vi "Add Data Tree.vi"(8 "error in (no error)":errorcluster, 11 "[V]System Tree View in":refnum<class "[V]System Tree View.lvclass">) -> (0 "error out":errorcluster, 3 "[V]System Tree View out":refnum<class "[V]System Tree View.lvclass">)   [LabVIEW 2020]
uses:
  <vilib>/HUASUI/Tree/Item/Type Definitions/Item Map.ctl
  <vilib>/HUASUI/Tree/Item/Item.lvclass
  <vilib>/HUASUI/Tree/Tree Helper/Tree Helper.lvclass
  <vilib>/HUASUI/Tree/Tree Helper.lvlib
  Models/Data List/Data List.lvclass
  [V]System Tree View.lvclass
  C:/Program Files (x86)/National Instruments/LabVIEW 2020/vi.lib/ActorFramework/Actor/Actor.lvclass
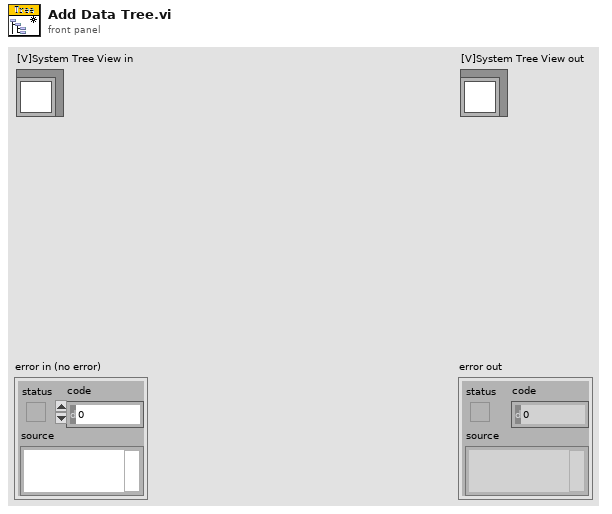
[diagram p1: front panel]
types:
  T1 = typedef "Tree Helper.lvlib/Item.lvclass/Item Map.ctl" = cluster{"Self Tag":string, "Parent Tag":string, "LeftCell Value":string, "RightCells Value":string[], "Is Child":bool, "Symbol Index":i32}
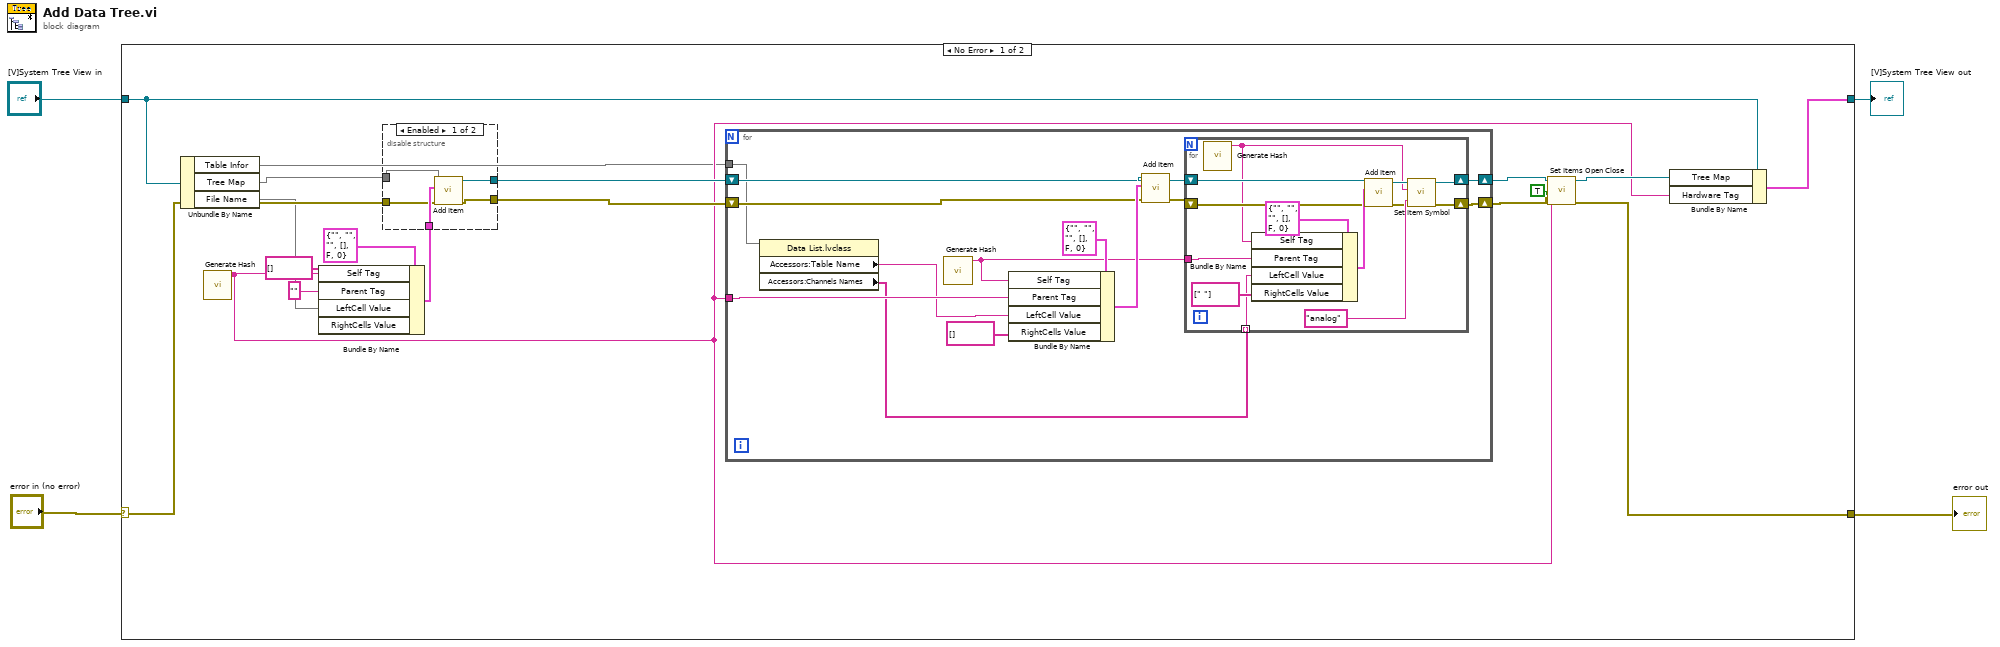
[diagram p0: block diagram]
diagram:
  n1 = case shown="No Error" "error in (no error)" {
    selector: "error in (no error)" -> [w15 w58]
    tunnel: [w7 w58] -> w3
    tunnel: [w21 w57] -> w1
    tunnel: "[V]System Tree View in" -> [w22 w57]
    frame No Error {
      n2 = Unbundle By Name(w22) -> ("Table Infor"=w6, "Tree Map"=w20, "File Name"=w5)
      n3 = call <vilib>:"Generate Hash.vi"() -> ("Hash"=w10:string)  [unwired: 10 in, 1 out]
      n4 = Bundle By Name(cluster=T1 {"Self Tag"="", "Parent Tag"="", "LeftCell Value"="", "RightCells Value"=[], "Is Child"=FALSE, "Symbol Index"=0} ("Item Map"), "Self Tag"=w10, "Parent Tag"="", "LeftCell Value"=w5, "RightCells Value"=string[] []) -> (w17:T1)
      n5 = disable-structure shown="Enabled" {
        disable-tunnel: w20 -> [w54 w56]
        disable-tunnel: [w53 w56] -> w19
        disable-tunnel: w17 -> [w52 _]
        disable-tunnel: w15 -> [w51 w55]
        disable-tunnel: [w50 w55] -> w14
        frame Enabled {
          n6 = call <vilib>:"Add Item.vi"("error in (no error)"=w51, "Item Map"=w52, "Tree Map in"=w54) -> ("error out"=w50:errorcluster, "Tree Map out"=w53:refnum<class "Tree Helper.lvclass">)  [unwired: 7 in]
        }
        frame Disabled {
        }
      }
      n7 = for {
        tunnel: w10 -> [w27]
        shift-right: [w28] -> w12
        shift-left: w19 -> [w30]
        shift-right: [w26] -> w8
        shift-left: w14 -> [w29]
        tunnel: w6 -> [w25]
        n8 = property class="Data List.lvclass"(reference=w25) -> ("Accessors:Table Name"=w24:string, "Accessors:Channels Names"=w23:string[])  [unwired: 1 in, 2 out]
        n9 = call <vilib>:"Generate Hash.vi"() -> ("Hash"=w31:string)  [unwired: 10 in, 1 out]
        n10 = Bundle By Name(cluster=T1 {"Self Tag"="", "Parent Tag"="", "LeftCell Value"="", "RightCells Value"=[], "Is Child"=FALSE, "Symbol Index"=0} ("Item Map"), "Self Tag"=w31, "Parent Tag"=w27, "LeftCell Value"=w24, "RightCells Value"=string[] []) -> (w33:T1)
        n11 = call <vilib>:"Add Item.vi"("error in (no error)"=w29, "Item Map"=w33, "Tree Map in"=w30) -> ("error out"=w35:errorcluster, "Tree Map out"=w36:refnum<class "Tree Helper.lvclass">)  [unwired: 7 in]
        n12 = for {
          shift-right: [w47] -> w28
          shift-left: w36 -> [w48]
          tunnel: w23 -> [w43] mode=indexing
          shift-right: [w41] -> w26
          shift-left: w35 -> [w40]
          tunnel: w31 -> [w39]
          n13 = call <vilib>:"Generate Hash.vi"() -> ("Hash"=w38:string)  [unwired: 10 in, 1 out]
          n14 = Bundle By Name(cluster=T1 {"Self Tag"="", "Parent Tag"="", "LeftCell Value"="", "RightCells Value"=[], "Is Child"=FALSE, "Symbol Index"=0} ("Item Map"), "Self Tag"=w38, "Parent Tag"=w39, "LeftCell Value"=w43, "RightCells Value"=string[] [" "]) -> (w45:T1)
          n15 = call <vilib>:"Add Item.vi"("error in (no error)"=w40, "Item Map"=w45, "Tree Map in"=w48) -> ("error out"=w37:errorcluster, "Tree Map out"=w49:refnum<class "Tree Helper.lvclass">)  [unwired: 7 in]
          n16 = call <vilib>:"Set Item Symbol.vi"("IconName"="analog", "error in (no error)"=w37, "Tag"=w38, "Tree Map in"=w49) -> ("error out"=w41:errorcluster, "Tree Map out"=w47:refnum<class "Tree Helper.lvclass">)  [unwired: 6 in]
        }
      }
      n17 = call <vilib>:"Set Items Open Close.vi"("error in (no error)"=w8, "Open?"=TRUE, "Tag"=w10, "Tree Map in"=w12) -> ("error out"=w7:errorcluster, "Tree Map out"=w11:refnum<class "Tree Helper.lvclass">)  [unwired: 6 in]
      n18 = Bundle By Name(cluster=w22, "Tree Map"=w11, "Hardware Tag"=w10) -> (w21:cluster{})
    }
    frame Error {
    }
  }
  "error out" <- w3
  "[V]System Tree View out" <- w1
